vi "Enertool final com fecho do dia.vi"() -> ()   [LabVIEW 2017]
uses:
  System.Windows.Forms
  <vilib>/addons/database/Connection.llb/DB Tools Open Connec (Path).vi
  <vilib>/addons/database/NI_Database_API.lvlib
panel:
  out "?":string
  in  "OApa 3":bool
  in  "OK Hora 2":bool
  out "Array 2":string[][](array[string])
  in  "OK Hora Mes 2":bool
  in  "?":bool
  in  "OK Hora Mes":bool
  out "Array":string[][](array[string])
  in  "stop":bool
  out "TabGeral":T1(tab)
  in  "Login":string
  in  "?":bool
  in  "Zapcine":bool
  in  "Banco Bic":bool
  in  "wammo":bool
  in  "Candando":bool
  in  "MENU":bool
  out "Tab Control":enum32{"ONLINE", "REPORT"}(tab)
  out "PT Hiper - Contagem Energia Reactiva GG":string
  out "PT Hiper - Energia Reactiva Total (MWh)":string
  out "PT Hiper - Energia Activa Total":string
  out "PT Hiper - Contagem Energia GG":string
  out "PT Hiper - Contagem Energia Rede":string
  out "PT Hiper - Contagem Energia Reactiva Rede":string
  in  "REPORT":bool
  out "?":enum32{"DIARIO", "MENSAL", "ANUAL"}(tab)
  out "Total Mês":dbl[](graph)
  out "?":string
  out "?":string
  out "Total Mês":dbl[](graph)
  out "Ano":string
  in  "Month Calendar .NET Control":refnum<k24>(container)
  in  "Periodo":string(combo)
  in  "Pesquisar":bool
  out "Consumo Total (MWh)":dbl
  in  "ONLINE":bool
  in  "Combo Box":string(combo)="Contagem de Energia Reactiva GG"
  out "Tab Control 2":enum32{"ONLINE", "REPORT"}(tab)
  out "PT Cinemas - Contagem Energia Rede":string
  out "PT Cinemas - Contagem Energia GG":string
  out "PT Cinemas - Energia Activa Total":string
  out "PT Cinemas - Energia Reactiva Total (MWh)":string
  out "PT Cinemas - Contagem Energia Reactiva Rede":string
  out "PT Cinemas - Contagem Energia Reactiva GG":string
  in  "REPORT 2":bool
  out "?":enum32{"DIARIO", "MENSAL", "ANUAL"}(tab)
  out "Total Mês":dbl[](graph)
  out "?":string
  out "?":string
  out "Total Mês":dbl[](graph)
  out "Ano 2":string
  in  "Month Calendar .NET Control 2":refnum<k24>(container)
  in  "Periodo 2":string(combo)
  in  "Pesquisar 2":bool
  out "Consumo Total (MWh) 2":dbl
  in  "Combo Box 2":string(combo)="Contagem de Energia Reactiva GG"
  in  "MENU 2":bool
  in  "OK Hora":bool
  in  "OApa 2":bool
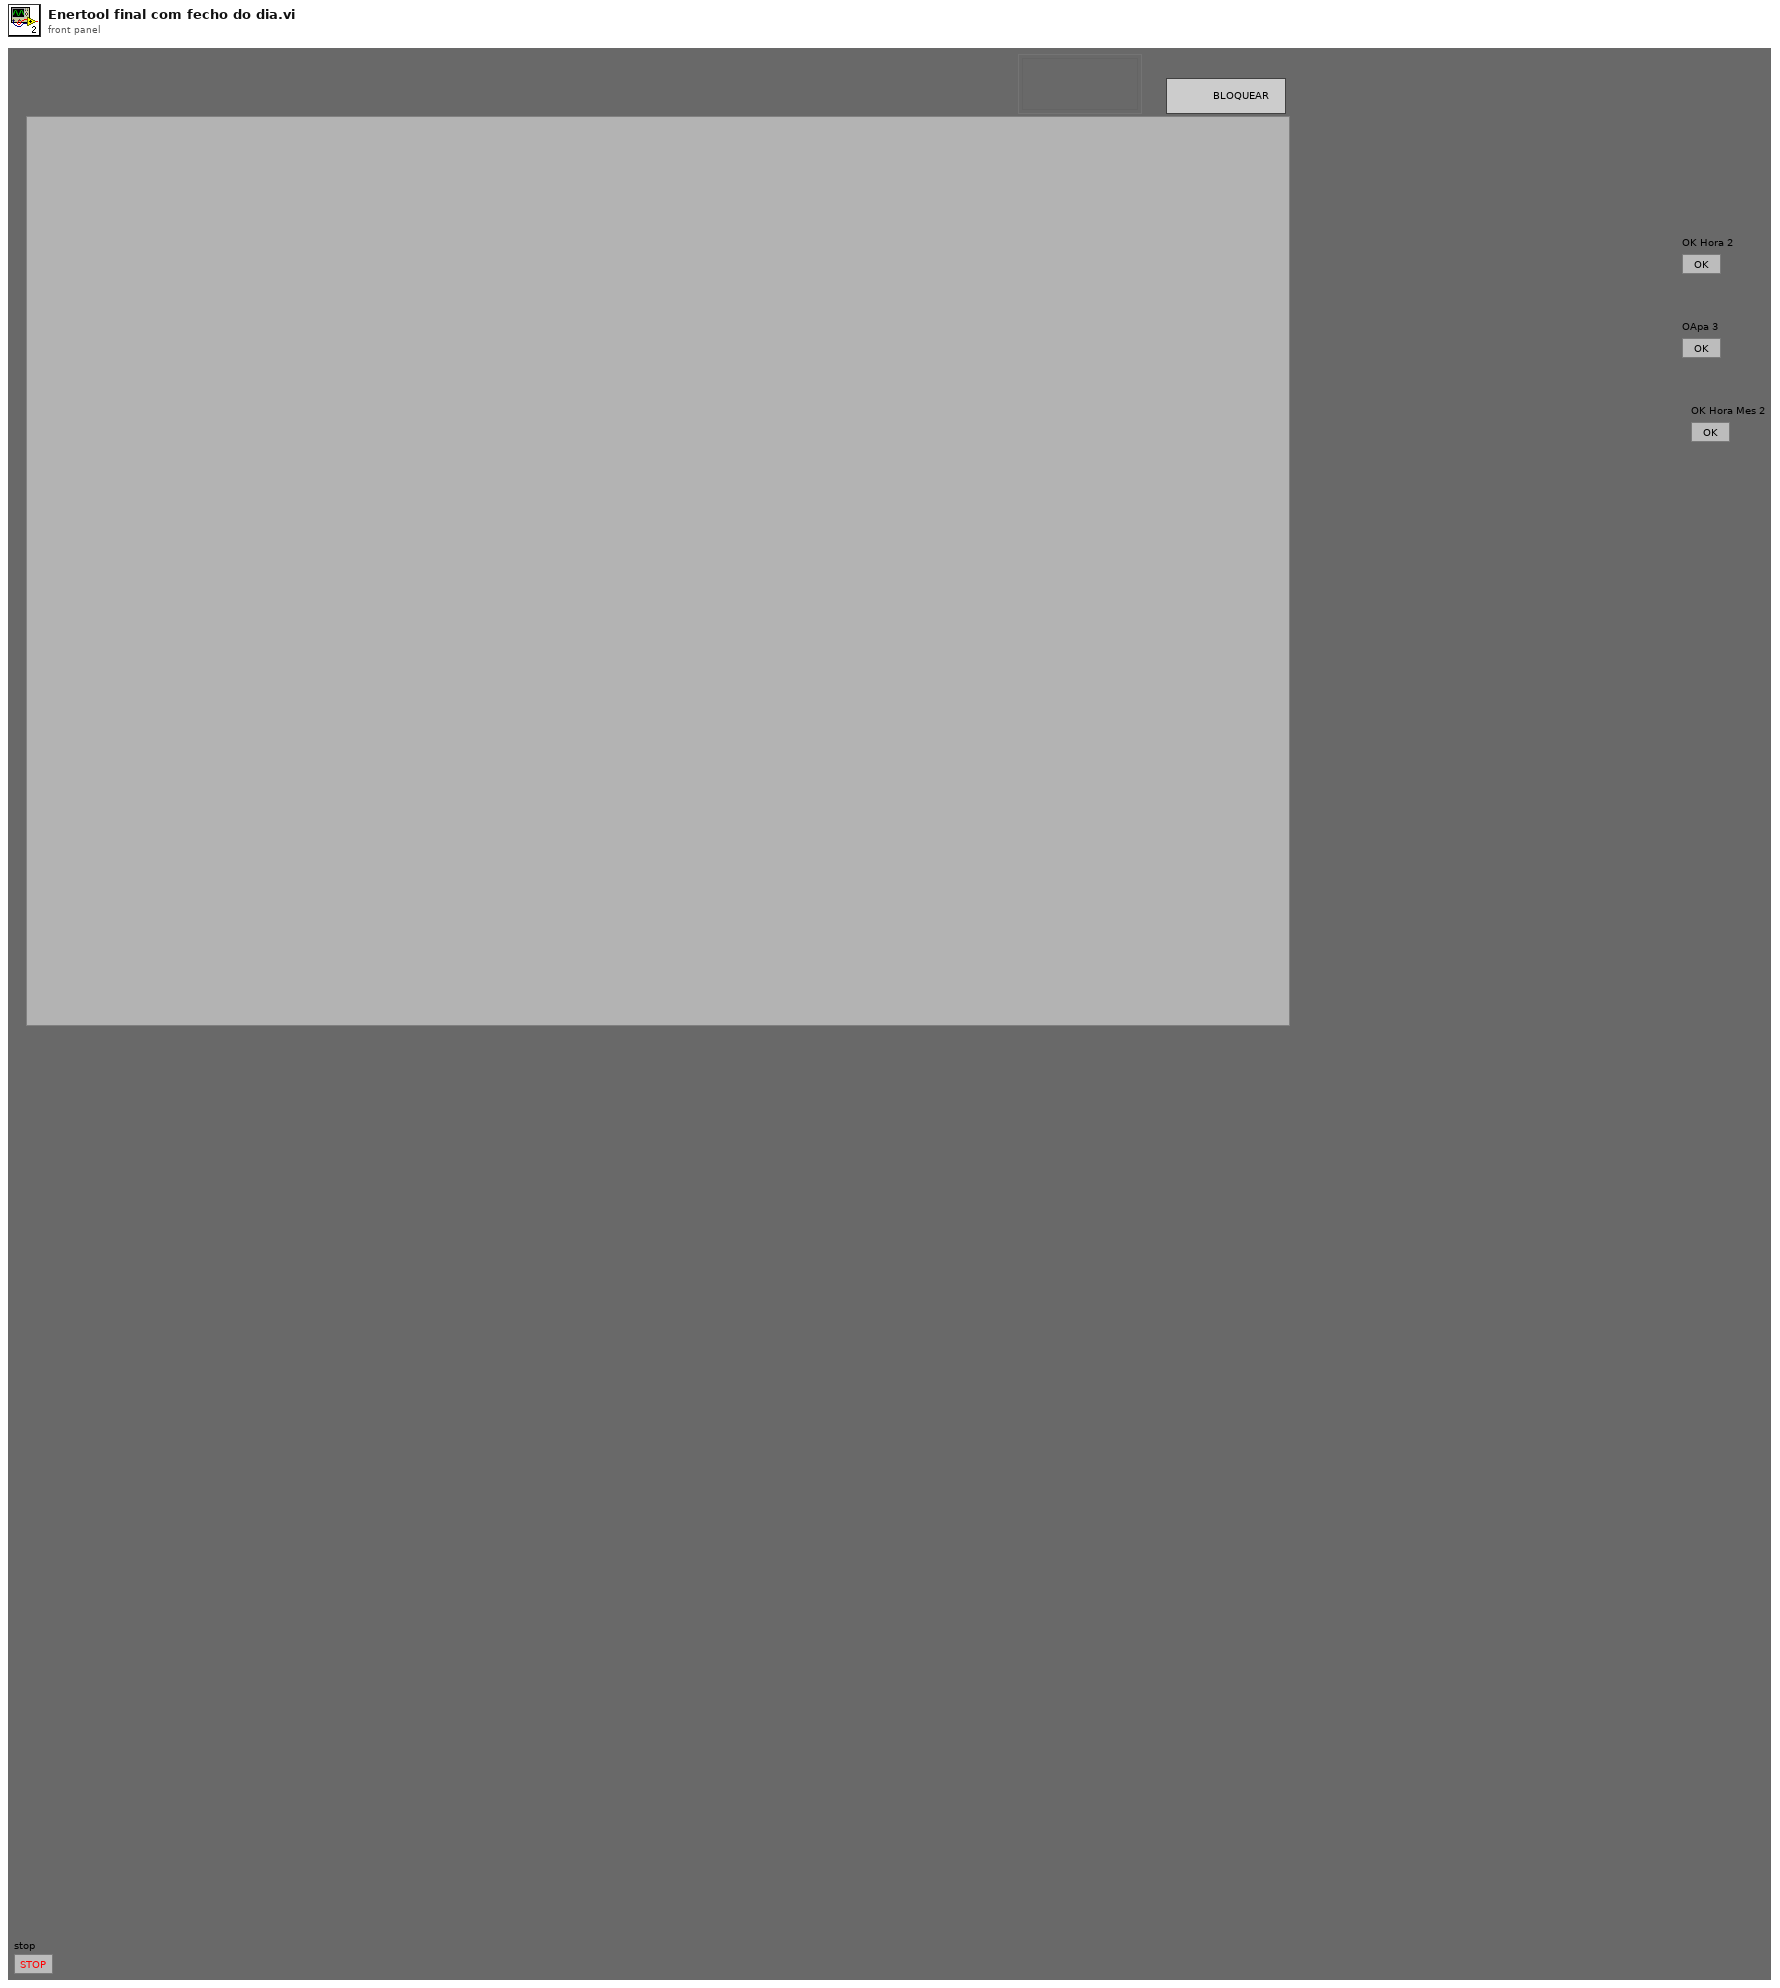
[diagram p1: front panel]
types:
  T1 = enum32{"Inicial", "Login", "Avennida", "HiperCandado", "ZapCinenma"}
  T2 = typedef "NI_Database_API.lvlib/Conn ObjectReference.ctl" = refnum<k1>
  T3 = enum16{"open", "replace", "create", "open or create", "replace or create", "replace or create with confirmation"}
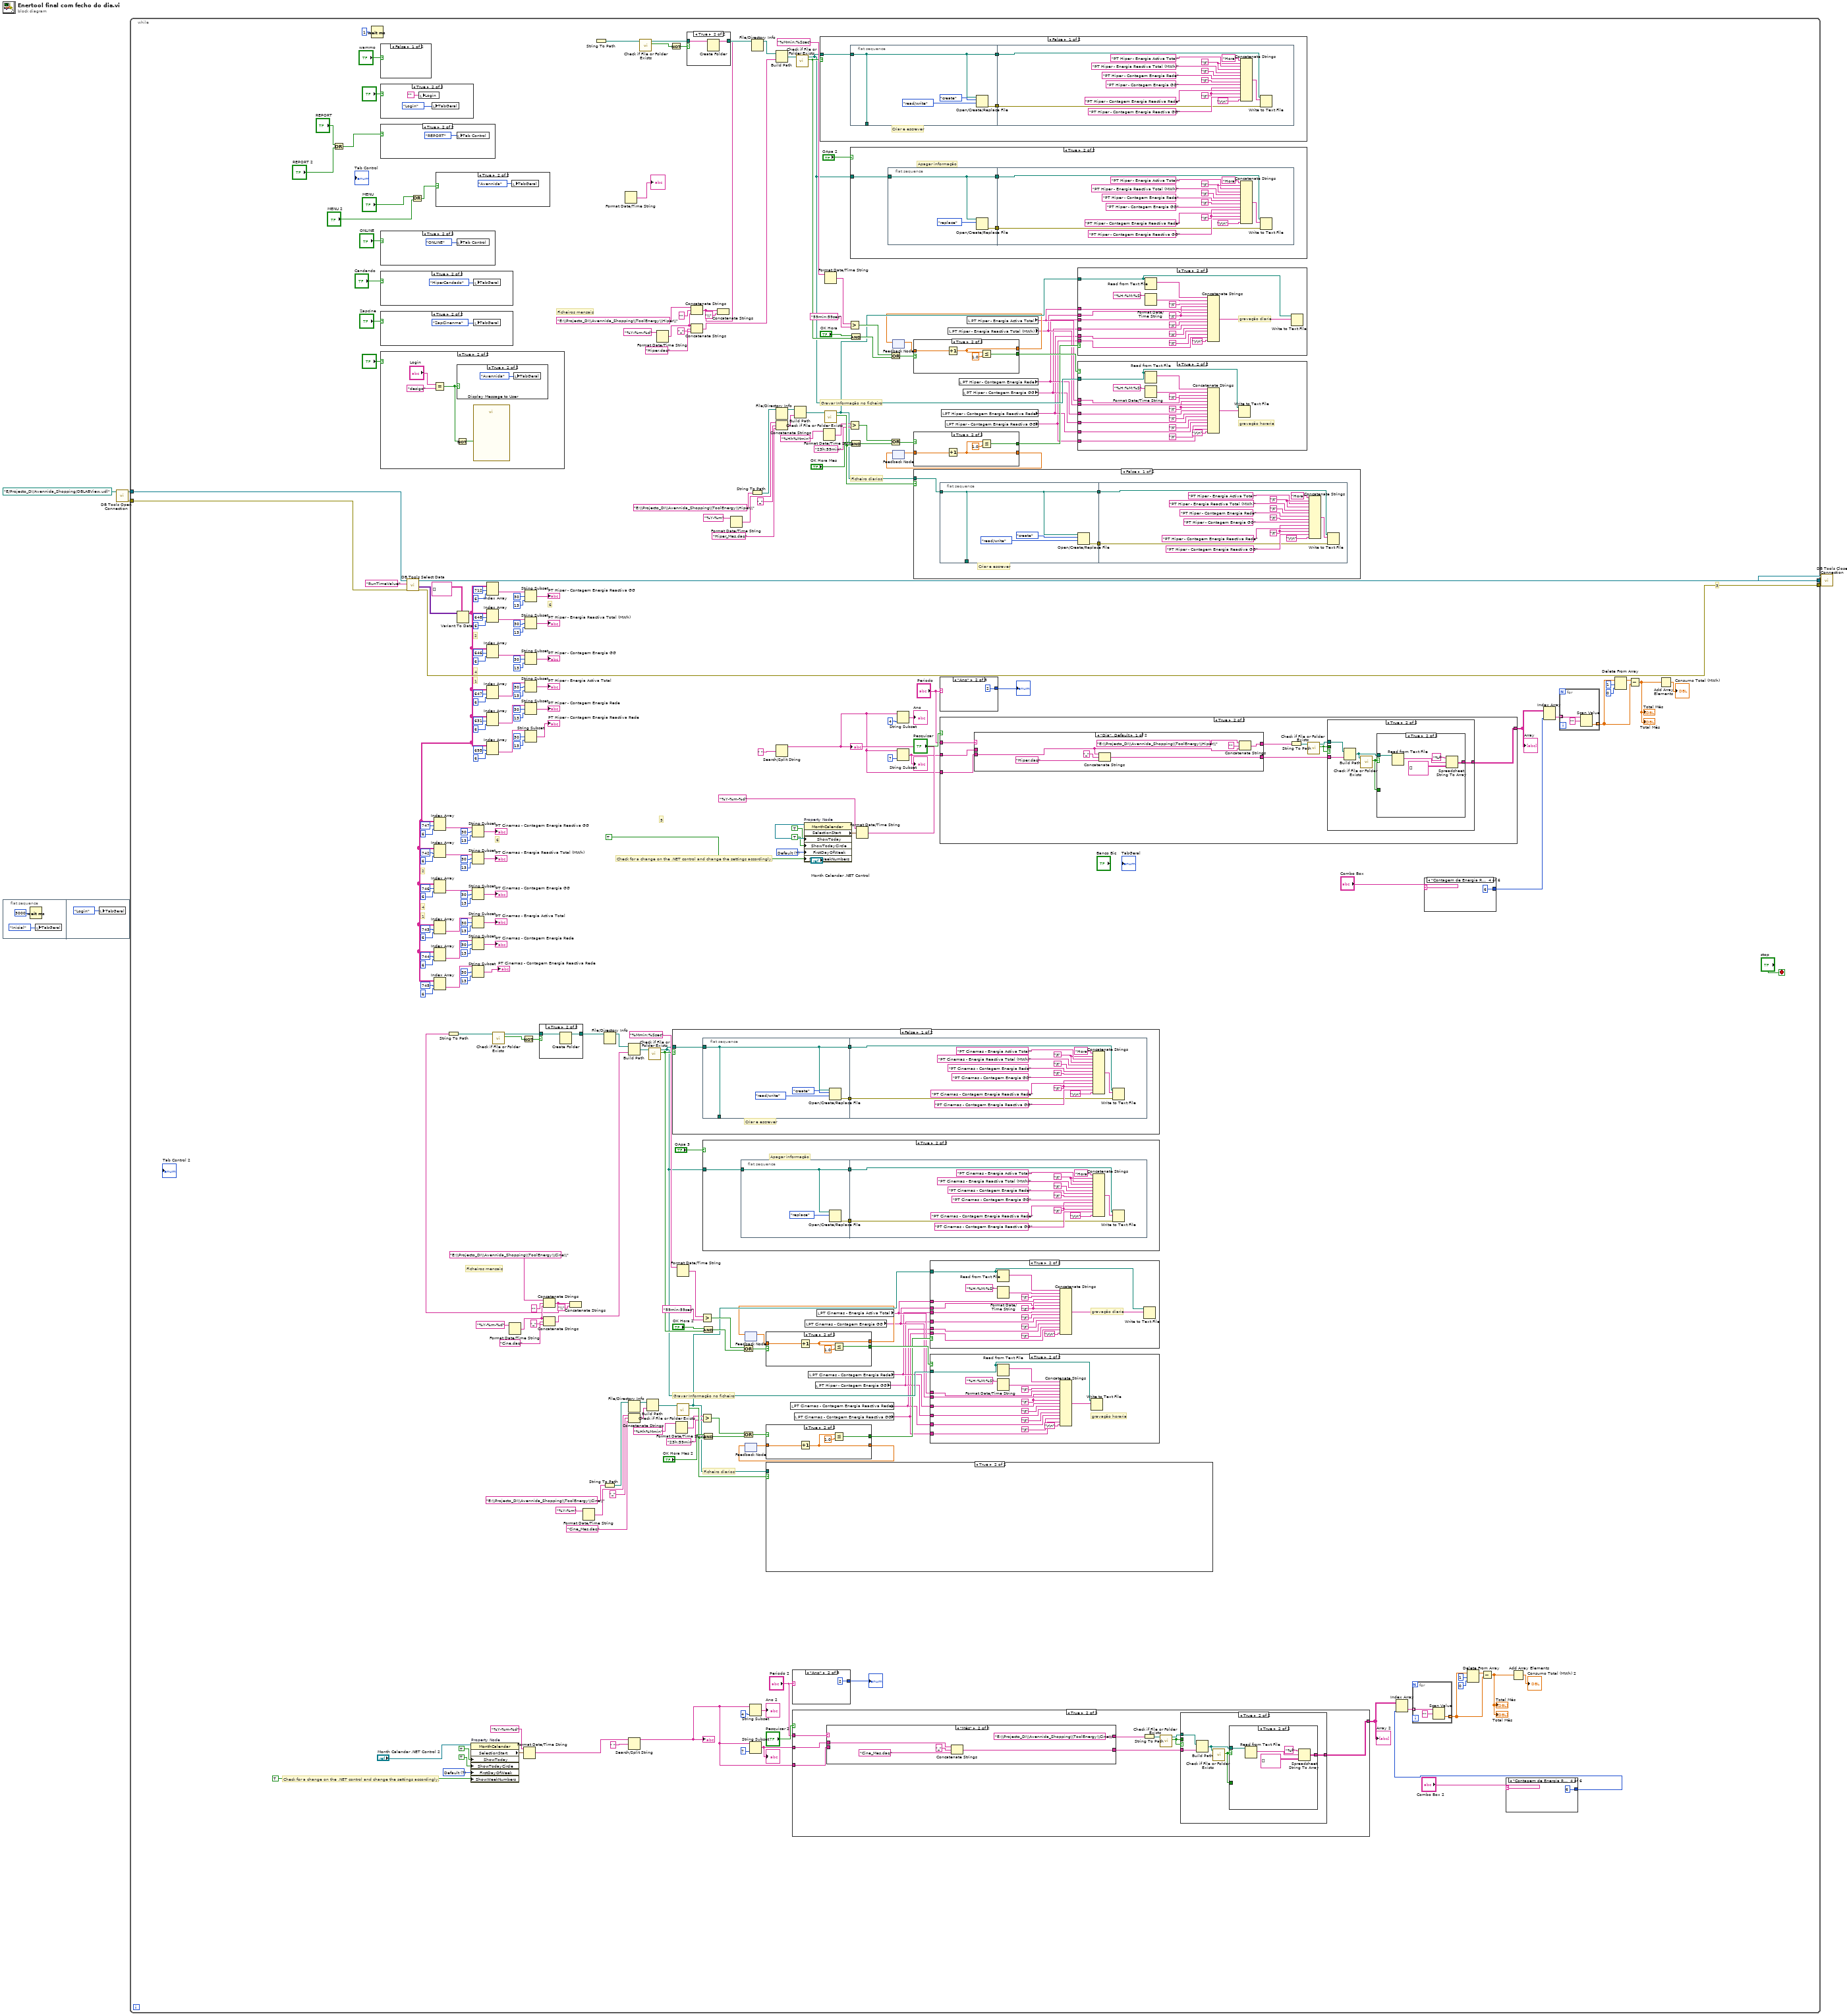
[diagram p0: block diagram]
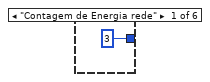
[diagram p2: hidden frame]
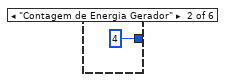
[diagram p3: hidden frame]
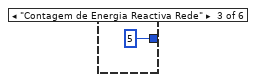
[diagram p4: hidden frame]
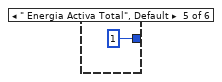
[diagram p5: hidden frame]
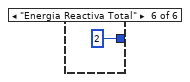
[diagram p6: hidden frame]
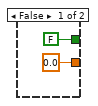
[diagram p7: hidden frame]
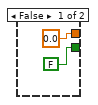
[diagram p8: hidden frame]
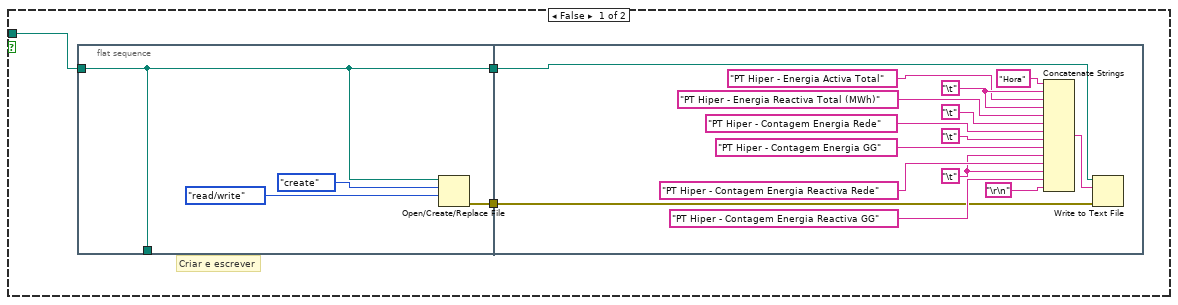
[diagram p11: hidden frame]
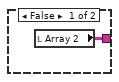
[diagram p14: hidden frame]
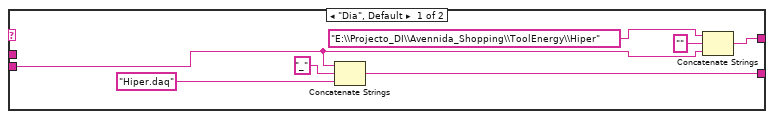
[diagram p15: hidden frame]
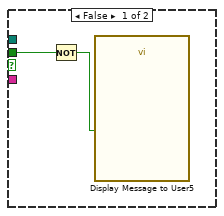
[diagram p16: hidden frame]
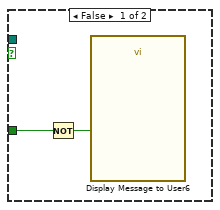
[diagram p17: hidden frame]
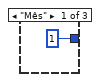
[diagram p18: hidden frame]
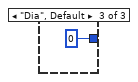
[diagram p19: hidden frame]
diagram:
  n1 = flat-sequence {
    frame #0 {
      n2 = Wait (ms)(milliseconds to wait=u32 3000) -> ()  [unwired: 1 out]
      n3 = local write "TabGeral"(T1."Inicial" ("TabGeral")) -> ()
    }
    frame #1 {
      n4 = local write "TabGeral"(T1."Login" ("TabGeral")) -> ()
    }
  }
  n5 = call-poly <vilib>:"DB Tools Open Connection.vi"("connection information"=path "E:/Projecto_DI/Avennida_Shopping/DBLABView.udl") -> ("error out"=w4:errorcluster, "connection reference"=w3:T2)  [unwired: 7 in]
  n6 = while {
    tunnel: w4 -> [w173]
    tunnel: w3 -> [w172]
    tunnel: [w171] -> w2
    tunnel: [w170] -> w1
    stop <- "stop" stop-if-true
    w93 = 7 items=["Monday", "Tuesday", "Wednesday", "Thursday", "Friday", "Saturday", "Sunday", "Default"] ("First Day of Week")
    w264 = 7 items=["Monday", "Tuesday", "Wednesday", "Thursday", "Friday", "Saturday", "Sunday", "Default"] ("First Day of Week")
    # "Ficheiros mensais"
    # "Ficheiro diarios"
    # "Gravar Informação no ficheiro"
    # "Check for a change on the .NET control and change the settings accordingly."
    # "1"
    # "2"
    # "4"
    # "6"
    # "1"
    # "2"
    # "3"
    # "4"
    # "5"
    # "6"
    # "Ficheiros mensais"
    # "Ficheiro diarios"
    # "Gravar Informação no ficheiro"
    # "Check for a change on the .NET control and change the settings accordingly."
    n7 = Or(x="REPORT", y="REPORT 2") -> (x .or. y?=w15:bool)
    n8 = Wait (ms)(milliseconds to wait=u32 1) -> ()  [unwired: 1 out]
    n9 = case shown="False" "wammo" {
      frame False {
      }
      frame True {
      }
    }
    n10 = case shown="True" "?" {
      frame False {
      }
      frame True {
        n11 = local write "Login"("") -> ()
        n12 = local write "TabGeral"(T1."Login" ("TabGeral")) -> ()
      }
    }
    n13 = case shown="True" w15 {
      frame False {
      }
      frame True {
        n14 = local write "Tab Control"(enum32{"ONLINE", "REPORT"}."REPORT" ("Tab Control")) -> ()
      }
    }
    n15 = case shown="True" "ONLINE" {
      frame False {
      }
      frame True {
        n16 = local write "Tab Control"(enum32{"ONLINE", "REPORT"}."ONLINE" ("Tab Control")) -> ()
      }
    }
    n17 = case shown="True" "Candando" {
      frame False {
      }
      frame True {
        n18 = local write "TabGeral"(T1."HiperCandado" ("TabGeral")) -> ()
      }
    }
    n19 = case shown="True" "Zapcine" {
      frame False {
      }
      frame True {
        n20 = local write "TabGeral"(T1."ZapCinenma" ("TabGeral")) -> ()
      }
    }
    n21 = case shown="True" "?" {
      frame False {
      }
      frame True {
        n22 = Equal?(x="Login", y="desigo") -> (x = y?=w577:bool)
        n23 = Not(x=w577) -> (.not. x?=w578:bool)
        n24 = case shown="True" w577 {
          frame False {
          }
          frame True {
            n25 = local write "TabGeral"(T1."Avennida" ("TabGeral")) -> ()
          }
        }
        n26 = call "Display Message to User"("Enable"=w578) -> ()  [unwired: 9 in, 2 out]
      }
    }
    n27 = call <vilib>:"DB Tools Select Data.vi"("error in (no error)"=w173, "table"="RunTimeValue", "connection reference"=w172) -> ("error out"=w171:errorcluster, "data"=w186:variant[][], "connection reference out"=w170:T2)  [unwired: 3 in]
    n28 = Or(x="MENU", y="MENU 2") -> (x .or. y?=w10:bool)
    n29 = case shown="True" w10 {
      frame False {
      }
      frame True {
        n30 = local write "TabGeral"(T1."Avennida" ("TabGeral")) -> ()
      }
    }
    n31 = Variant To Data(type=string[][] [], Variant=w186) -> (data=w99:string[][])  [unwired: 1 in, 1 out]
    n32 = Index Array(array=w99, index (row)=747, index (col)=6 ("disabled index (col) 2")) -> (element=w114:string)
    n33 = Index Array(array=w99, index (row)=742, index (col)=6 ("disabled index (col) 3")) -> (element=w127:string)
    n34 = Index Array(array=w99, index (row)=746, index (col)=6 ("disabled index (col) 3")) -> (element=w123:string)
    n35 = Index Array(array=w99, index (row)=743, index (col)=6 ("disabled index (col) 4")) -> (element=w119:string)
    n36 = Index Array(array=w99, index (row)=744, index (col)=6 ("disabled index (col) 3")) -> (element=w134:string)
    n37 = Index Array(array=w99, index (row)=745, index (col)=6 ("disabled index (col)")) -> (element=w116:string)
    n38 = property on="Property Node" class="MonthCalendar"(reference="Month Calendar .NET Control 2", "ShowToday"=TRUE ("Show Today"), "ShowTodayCircle"=TRUE ("Show Today Circle"), "FirstDayOfWeek"=w93, "ShowWeekNumbers"=TRUE ("Show Week Numbers")) -> ("SelectionStart"=w95:timestamp)  [unwired: 1 in, 2 out]
    n39 = String Subset(string=w114, offset (0)=30, length (rest)=13 ("length (rest)")) -> (substring=→"PT Cinemas - Contagem Energia Reactiva GG":string)
    n40 = String Subset(string=w127, offset (0)=30, length (rest)=13 ("length (rest)")) -> (substring=→"PT Cinemas - Energia Reactiva Total (MWh)":string)
    n41 = String Subset(string=w123, offset (0)=30, length (rest)=13 ("length (rest)")) -> (substring=→"PT Cinemas - Contagem Energia GG":string)
    n42 = String Subset(string=w119, offset (0)=30, length (rest)=13 ("length (rest)")) -> (substring=→"PT Cinemas - Energia Activa Total":string)
    n43 = String Subset(string=w134, offset (0)=30, length (rest)=13 ("length (rest)")) -> (substring=→"PT Cinemas - Contagem Energia Rede":string)
    n44 = String Subset(string=w116, offset (0)=30, length (rest)=13 ("length (rest)")) -> (substring=→"PT Cinemas - Contagem Energia Reactiva Rede":string)
    n45 = Index Array(array=w99, index (row)=712, index (col)=6 ("disabled index (col) 2")) -> (element=w165:string)
    n46 = Index Array(array=w99, index (row)=648, index (col)=6 ("disabled index (col) 3")) -> (element=w152:string)
    n47 = Index Array(array=w99, index (row)=646, index (col)=6 ("disabled index (col) 3")) -> (element=w156:string)
    n48 = Index Array(array=w99, index (row)=647, index (col)=6 ("disabled index (col) 4")) -> (element=w160:string)
    n49 = Index Array(array=w99, index (row)=631, index (col)=6 ("disabled index (col) 3")) -> (element=w145:string)
    n50 = Index Array(array=w99, index (row)=695, index (col)=6 ("disabled index (col)")) -> (element=w163:string)
    n51 = Format Date/Time String(time format string (%c)="%Y-%m-%d") -> (date/time string=w59:string)  [unwired: 2 in]
    n52 = Format Date/Time String(time format string (%c)="%Y-%m-%d", seconds (now)=w95) -> (date/time string=w94:string)  [unwired: 1 in]
    n53 = String Subset(string=w165, offset (0)=30, length (rest)=13 ("length (rest)")) -> (substring=→"PT Hiper - Contagem Energia Reactiva GG":string)
    n54 = String Subset(string=w152, offset (0)=30, length (rest)=13 ("length (rest)")) -> (substring=→"PT Hiper - Energia Reactiva Total (MWh)":string)
    n55 = String Subset(string=w156, offset (0)=30, length (rest)=13 ("length (rest)")) -> (substring=→"PT Hiper - Contagem Energia GG":string)
    n56 = String Subset(string=w160, offset (0)=30, length (rest)=13 ("length (rest)")) -> (substring=→"PT Hiper - Energia Activa Total":string)
    n57 = String Subset(string=w145, offset (0)=30, length (rest)=13 ("length (rest)")) -> (substring=→"PT Hiper - Contagem Energia Rede":string)
    n58 = String Subset(string=w163, offset (0)=30, length (rest)=13 ("length (rest)")) -> (substring=→"PT Hiper - Contagem Energia Reactiva Rede":string)
    n59 = Concatenate Strings("E:\\Projecto_DI\\Avennida_Shopping\\ToolEnergy\\Cine\\", "" ("string"), w59) -> (w48:string)
    n60 = String To Path(string=w48) -> (path=w50:path)
    n61 = call <vilib>:"Check if File or Folder Exists.vi"("path"=w50) -> ("file or folder exists?"=w52:bool, "dup path"=w51:path)  [unwired: 8 in, 1 out]
    n62 = Not(x=w52) -> (.not. x?=w53:bool)
    n63 = case shown="True" w53 {
      tunnel: w51 -> [w366 w368]
      tunnel: [w366 w367] -> w54
      frame False {
      }
      frame True {
        n64 = Create Folder(path (use dialog)=w368) -> (created path=w367:path)  [unwired: 2 in, 2 out]
      }
    }
    n65 = Concatenate Strings(w59, "_" ("string"), "Cine.daq" ("name or relative path")) -> (w58:string)
    n66 = Concatenate Strings(w48, "\\") -> ()  [unwired: 1 out]
    n67 = Format Date/Time String(time format string (%c)="%Y-%m") -> (date/time string=w43:string)  [unwired: 2 in]
    n68 = String To Path(string="E:\\Projecto_DI\\Avennida_Shopping\\ToolEnergy\\Cine\\") -> (path=w37:path)
    n69 = File/Directory Info(path=w54) -> (path out=w55:path)  [unwired: 1 in, 6 out]
    n70 = Format Date/Time String() -> (date/time string=→"?":string)  [unwired: 3 in]
    n71 = Build Path(base path=w55, name or relative path=w58) -> (appended path=w56:path)
    n72 = File/Directory Info(path=w37) -> (path out=w39:path)  [unwired: 1 in, 6 out]
    n73 = Concatenate Strings(w43, "_" ("string"), "Cine_Mes.daq" ("name or relative path")) -> (w42:string)
    n74 = Search/Split String(string=w94, search string/char (-)=" ") -> (substring before match=w83:string)  [unwired: 1 in, 2 out]
    "?" <- w83
    n75 = Build Path(base path=w39, name or relative path=w42) -> (appended path=w40:path)
    n76 = call <vilib>:"Check if File or Folder Exists.vi"("path"=w56) -> ("file or folder exists?"=w46:bool, "dup path"=w45:path)  [unwired: 8 in, 1 out]
    n77 = Format Date/Time String(time format string (%c)="%Y-%m-%d") -> (date/time string=w223:string)  [unwired: 2 in]
    n78 = case shown="False" w46 {
      tunnel: w45 -> [w346 _]
      frame False {
        # "Criar e escrever"
        n79 = flat-sequence {
          tunnel: w346 -> [w348]
          tunnel: [w348] -> _
          tunnel: [w348] -> w345
          tunnel: [w347] -> w344
          tunnel: w345 -> [w351]
          tunnel: w344 -> [w352]
          frame #0 {
            n80 = Open/Create/Replace File(file path (use dialog)=w348, operation (0:open)=T3."create", access (0:read/write)=enum16{"read/write", "read-only", "write-only"}."read/write") -> (error out=w347:errorcluster)  [unwired: 3 in, 2 out]
          }
          frame #1 {
            w362 = "\t"
            w355 = "\t"
            n81 = Concatenate Strings("Hora" ("string"), w355, "PT Cinemas - Energia Activa Total" ("string"), w355, "PT Cinemas - Energia Reactiva Total (MWh)" ("string"), "\t", "PT Cinemas - Contagem Energia Rede" ("string"), "\t", "PT Cinemas - Contagem Energia GG" ("string"), w362, "PT Cinemas - Contagem Energia Reactiva Rede" ("string"), w362, "PT Cinemas - Contagem Energia Reactiva GG" ("string"), "\r\n") -> (w353:string)
            n82 = Write to Text File(file (use dialog)=w351, text=w353, error in=w352) -> ()  [unwired: 1 in, 3 out]
          }
        }
      }
      frame True {
      }
    }
    n83 = Format Date/Time String(time format string (%c)="%Hh%Mmin") -> (date/time string=w67:string)  [unwired: 2 in]
    n84 = call <vilib>:"Check if File or Folder Exists.vi"("path"=w40) -> ("file or folder exists?"=w73:bool, "dup path"=w35:path)  [unwired: 8 in, 1 out]
    n85 = Format Date/Time String(time format string (%c)="%Mmin:%Ssec") -> (date/time string=w71:string)  [unwired: 2 in]
    n86 = Concatenate Strings("E:\\Projecto_DI\\Avennida_Shopping\\ToolEnergy\\Hiper\\", "" ("string"), w223) -> (w212:string)
    n87 = String To Path(string=w212) -> (path=w214:path)
    n88 = call <vilib>:"Check if File or Folder Exists.vi"("path"=w214) -> ("file or folder exists?"=w216:bool, "dup path"=w215:path)  [unwired: 8 in, 1 out]
    n89 = Not(x=w216) -> (.not. x?=w217:bool)
    n90 = case shown="True" w217 {
      tunnel: w215 -> [w527 w529]
      tunnel: [w527 w528] -> w218
      frame False {
      }
      frame True {
        n91 = Create Folder(path (use dialog)=w529) -> (created path=w528:path)  [unwired: 2 in, 2 out]
      }
    }
    n92 = Concatenate Strings(w223, "_" ("string"), "Hiper.daq" ("name or relative path")) -> (w222:string)
    n93 = Greater?(x=w71, y="59min:59sec") -> (0:w68:bool)
    n94 = Greater?(x=w67, y="23h:59min" ("y 2")) -> (0:w64:bool)
    n95 = And(x="OK Hora 2", y=w46) -> (x .and. y?=w69:bool)
    n96 = And(x="OK Hora Mes 2", y=w73) -> (x .and. y?=w65:bool)
    n97 = case shown="True" "OApa 3" {
      tunnel: w45 -> [_ w413]
      frame False {
      }
      frame True {
        # "Apagar informação"
        n98 = flat-sequence {
          tunnel: w413 -> [w414]
          tunnel: [w415] -> w412
          tunnel: [w414] -> w411
          tunnel: w412 -> [w418]
          tunnel: w411 -> [w417]
          frame #0 {
            n99 = Open/Create/Replace File(file path (use dialog)=w414, operation (0:open)=T3."replace") -> (error out=w415:errorcluster)  [unwired: 4 in, 2 out]
          }
          frame #1 {
            w422 = "\t"
            w429 = "\t"
            n100 = Concatenate Strings("Hora" ("string"), w429, "PT Cinemas - Energia Activa Total" ("string"), w429, "PT Cinemas - Energia Reactiva Total (MWh)" ("string"), "\t", "PT Cinemas - Contagem Energia Rede" ("string"), "\t", "PT Cinemas - Contagem Energia GG" ("string"), w422, "PT Cinemas - Contagem Energia Reactiva Rede" ("string"), w422, "PT Cinemas - Contagem Energia Reactiva GG" ("string"), "\r\n") -> (w431:string)
            n101 = Write to Text File(file (use dialog)=w417, text=w431, error in=w418) -> ()  [unwired: 1 in, 3 out]
          }
        }
      }
    }
    n102 = Concatenate Strings(w212, "\\") -> ()  [unwired: 1 out]
    n103 = Format Date/Time String(time format string (%c)="%Y-%m") -> (date/time string=w207:string)  [unwired: 2 in]
    n104 = Or(x=w68, y=w69) -> (x .or. y?=w32:bool)
    n105 = Or(x=w64, y=w65) -> (x .or. y?=w27:bool)
    n106 = feedback #1() -> (w33:dbl)  [unwired: 1 in]
    n107 = feedback #2() -> (w28:dbl)  [unwired: 1 in]
    n108 = String Subset(string=w83, length (rest)=4 ("length (rest)")) -> (substring=→"Ano 2":string)  [unwired: 1 in]
    n109 = String Subset(string=w83, length (rest)=7 ("length (rest)")) -> (substring=w25:string)  [unwired: 1 in]
    "?" <- w25
    n110 = String To Path(string="E:\\Projecto_DI\\Avennida_Shopping\\ToolEnergy\\Hiper\\") -> (path=w201:path)
    n111 = File/Directory Info(path=w218) -> (path out=w219:path)  [unwired: 1 in, 6 out]
    n112 = case shown="True" w32 {
      tunnel: [0.0 w284] -> w34
      tunnel: w33 -> [_ w287]
      tunnel: [FALSE w286] -> w31
      frame False {
      }
      frame True {
        n113 = Increment(x=w287) -> (x+1=w284:dbl)
        n114 = Less Or Equal?(x=w284, y=1.0) -> (x <= y?=w286:bool)
      }
    }
    n115 = feedback-in #1(w34) -> ()
    n116 = case shown="True" w27 {
      tunnel: [0.0 w279] -> w30
      tunnel: [FALSE w281] -> w29
      tunnel: w28 -> [_ w278]
      frame False {
      }
      frame True {
        n117 = Increment(x=w278) -> (x+1=w279:dbl)
        n118 = Less Or Equal?(x=w279, y=1.0) -> (x <= y?=w281:bool)
      }
    }
    n119 = feedback-in #2(w30) -> ()
    n120 = case shown="True" w73 {
      tunnel: w35 -> [w322 _]
      frame False {
        # "Criar e escrever"
        n121 = flat-sequence {
          tunnel: w322 -> [w326]
          tunnel: [w326] -> _
          tunnel: [w326] -> w324
          tunnel: [w325] -> w323
          tunnel: w324 -> [w333]
          tunnel: w323 -> [w332]
          frame #0 {
            n122 = Open/Create/Replace File(file path (use dialog)=w326, operation (0:open)=T3."create", access (0:read/write)=enum16{"read/write", "read-only", "write-only"}."read/write") -> (error out=w325:errorcluster)  [unwired: 3 in, 2 out]
          }
          frame #1 {
            w337 = "\t"
            w330 = "\t"
            n123 = Concatenate Strings("Hora" ("string"), w330, "PT Hiper - Energia Activa Total" ("string"), w330, "PT Hiper - Energia Reactiva Total (MWh)" ("string"), "\t", "PT Hiper - Contagem Energia Rede" ("string"), "\t", "PT Hiper - Contagem Energia GG" ("string"), w337, "PT Hiper - Contagem Energia Reactiva Rede" ("string"), w337, "PT Hiper - Contagem Energia Reactiva GG" ("string"), "\r\n") -> (w334:string)
            n124 = Write to Text File(file (use dialog)=w333, text=w334, error in=w332) -> ()  [unwired: 1 in, 3 out]
          }
        }
      }
      frame True {
      }
    }
    n125 = Build Path(base path=w219, name or relative path=w222) -> (appended path=w220:path)
    n126 = File/Directory Info(path=w201) -> (path out=w203:path)  [unwired: 1 in, 6 out]
    n127 = Concatenate Strings(w207, "_" ("string"), "Hiper_Mes.daq" ("name or relative path")) -> (w206:string)
    n128 = local read "PT Cinemas - Contagem Energia Reactiva Rede"() -> (w19:string)
    n129 = case shown="\"Ano\"" "Periodo 2" {
      tunnel: [1 2 0] -> w85
      frame "Mês" {
      }
      frame "Ano" {
      }
      frame "Dia", Default {
      }
    }
    "?" <- w85
    n130 = case shown="True" "Pesquisar 2" {
      tunnel: w83 -> [_ w375]
      tunnel: [w369 w372] -> w81
      tunnel: "Periodo 2" -> [_ w371]
      tunnel: w25 -> [_ w370]
      frame False {
        n131 = local read "Array 2"() -> (w369:string[][])
      }
      frame True {
        n132 = case shown="\"Mês\"" w371 {
          tunnel: [w382 "E:\\Projecto_DI\\Avennida_Shopping\\ToolEnergy\\Cine\\"] -> w376
          tunnel: w375 -> [w380 _]
          tunnel: [w379 w388] -> w374
          tunnel: w370 -> [_ w386]
          frame "Dia", Default {
            n133 = Concatenate Strings(w380, "_" ("string"), "Hiper.daq" ("name or relative path")) -> (w379:string)
            n134 = Concatenate Strings("E:\\Projecto_DI\\Avennida_Shopping\\ToolEnergy\\Hiper", "" ("string"), w380) -> (w382:string)
          }
          frame "Mês" {
            n135 = Concatenate Strings(w386, "_" ("string"), "Cine_Mes.daq" ("name or relative path")) -> (w388:string)
          }
        }
        n136 = String To Path(string=w376) -> (path=w377:path)
        n137 = call <vilib>:"Check if File or Folder Exists.vi"("path"=w377) -> ("file or folder exists?"=w373:bool, "dup path"=w378:path)  [unwired: 8 in, 1 out]
        n138 = case shown="True" w373 {
          tunnel: w378 -> [_ w395]
          tunnel: w374 -> [_ w397]
          tunnel: w373 -> [w391 _]
          tunnel: [_ w394] -> w372
          frame False {
            n139 = Not(x=w391) -> (.not. x?=w392:bool)
            n140 = call "Display Message to User5"("Enable"=w392) -> ()  [unwired: 9 in, 2 out]
          }
          frame True {
            n141 = Build Path(base path=w395, name or relative path=w397) -> (appended path=w393:path)
            n142 = call <vilib>:"Check if File or Folder Exists.vi"("path"=w393) -> ("file or folder exists?"=w396:bool)  [unwired: 8 in, 2 out]
            n143 = case shown="True" w396 {
              tunnel: w396 -> [w398 _]
              tunnel: w393 -> [_ w401]
              tunnel: [_ w400] -> w394
              frame False {
                n144 = Not(x=w398) -> (.not. x?=w399:bool)
                n145 = call "Display Message to User6"("Enable"=w399) -> ()  [unwired: 9 in, 2 out]
              }
              frame True {
                n146 = Read from Text File(file (use dialog)=w401) -> (text=w404:string)  [unwired: 3 in, 3 out]
                n147 = Spreadsheet String To Array(format string="%f", spreadsheet string=w404, array type (2D Dbl)=string[][] [] ("Array")) -> (array=w400:string[][])  [unwired: 1 in]
              }
            }
          }
        }
      }
    }
    "Array 2" <- w81
    n148 = Build Path(base path=w203, name or relative path=w206) -> (appended path=w204:path)
    n149 = local read "PT Cinemas - Contagem Energia Reactiva GG"() -> (w18:string)
    n150 = call <vilib>:"Check if File or Folder Exists.vi"("path"=w220) -> ("file or folder exists?"=w210:bool, "dup path"=w209:path)  [unwired: 8 in, 1 out]
    n151 = property on="Property Node" class="MonthCalendar"(reference="Month Calendar .NET Control", "ShowToday"=TRUE ("Show Today"), "ShowTodayCircle"=TRUE ("Show Today Circle"), "FirstDayOfWeek"=w264, "ShowWeekNumbers"=TRUE ("Show Week Numbers")) -> ("SelectionStart"=w266:timestamp)  [unwired: 1 in, 2 out]
    n152 = local read "PT Cinemas - Contagem Energia GG"() -> (w22:string)
    n153 = local read "PT Cinemas - Contagem Energia Rede"() -> (w21:string)
    n154 = local read "PT Hiper - Contagem Energia GG"() -> (w20:string)
    n155 = local read "PT Cinemas - Energia Activa Total"() -> (w23:string)
    n156 = case shown="False" w210 {
      tunnel: w209 -> [w507 _]
      frame False {
        # "Criar e escrever"
        n157 = flat-sequence {
          tunnel: w507 -> [w509]
          tunnel: [w509] -> _
          tunnel: [w509] -> w506
          tunnel: [w508] -> w505
          tunnel: w506 -> [w512]
          tunnel: w505 -> [w513]
          frame #0 {
            n158 = Open/Create/Replace File(file path (use dialog)=w509, operation (0:open)=T3."create", access (0:read/write)=enum16{"read/write", "read-only", "write-only"}."read/write") -> (error out=w508:errorcluster)  [unwired: 3 in, 2 out]
          }
          frame #1 {
            w523 = "\t"
            w516 = "\t"
            n159 = Concatenate Strings("Hora" ("string"), w516, "PT Hiper - Energia Activa Total" ("string"), w516, "PT Hiper - Energia Reactiva Total (MWh)" ("string"), "\t", "PT Hiper - Contagem Energia Rede" ("string"), "\t", "PT Hiper - Contagem Energia GG" ("string"), w523, "PT Hiper - Contagem Energia Reactiva Rede" ("string"), w523, "PT Hiper - Contagem Energia Reactiva GG" ("string"), "\r\n") -> (w514:string)
            n160 = Write to Text File(file (use dialog)=w512, text=w514, error in=w513) -> ()  [unwired: 1 in, 3 out]
          }
        }
      }
      frame True {
      }
    }
    n161 = Format Date/Time String(time format string (%c)="%Hh%Mmin") -> (date/time string=w231:string)  [unwired: 2 in]
    n162 = call <vilib>:"Check if File or Folder Exists.vi"("path"=w204) -> ("file or folder exists?"=w237:bool, "dup path"=w199:path)  [unwired: 8 in, 1 out]
    n163 = Format Date/Time String(time format string (%c)="%Mmin:%Ssec") -> (date/time string=w235:string)  [unwired: 2 in]
    n164 = Greater?(x=w235, y="59min:59sec") -> (0:w232:bool)
    n165 = Greater?(x=w231, y="23h:59min" ("y 2")) -> (0:w228:bool)
    n166 = And(x="OK Hora", y=w210) -> (x .and. y?=w233:bool)
    n167 = And(x="OK Hora Mes", y=w237) -> (x .and. y?=w229:bool)
    n168 = case shown="True" "OApa 2" {
      tunnel: w209 -> [_ w587]
      frame False {
      }
      frame True {
        # "Apagar informação"
        n169 = flat-sequence {
          tunnel: w587 -> [w588]
          tunnel: [w589] -> w586
          tunnel: [w588] -> w585
          tunnel: w586 -> [w592]
          tunnel: w585 -> [w591]
          frame #0 {
            n170 = Open/Create/Replace File(file path (use dialog)=w588, operation (0:open)=T3."replace") -> (error out=w589:errorcluster)  [unwired: 4 in, 2 out]
          }
          frame #1 {
            w596 = "\t"
            w603 = "\t"
            n171 = Concatenate Strings("Hora" ("string"), w603, "PT Hiper - Energia Activa Total" ("string"), w603, "PT Hiper - Energia Reactiva Total (MWh)" ("string"), "\t", "PT Hiper - Contagem Energia Rede" ("string"), "\t", "PT Hiper - Contagem Energia GG" ("string"), w596, "PT Hiper - Contagem Energia Reactiva Rede" ("string"), w596, "PT Hiper - Contagem Energia Reactiva GG" ("string"), "\r\n") -> (w605:string)
            n172 = Write to Text File(file (use dialog)=w591, text=w605, error in=w592) -> ()  [unwired: 1 in, 3 out]
          }
        }
      }
    }
    n173 = Format Date/Time String(time format string (%c)="%Y-%m-%d", seconds (now)=w266) -> (date/time string=w265:string)  [unwired: 1 in]
    n174 = Search/Split String(string=w265, search string/char (-)=" ") -> (substring before match=w251:string)  [unwired: 1 in, 2 out]
    "?" <- w251
    n175 = Or(x=w232, y=w233) -> (x .or. y?=w196:bool)
    n176 = Or(x=w228, y=w229) -> (x .or. y?=w191:bool)
    n177 = feedback #3() -> (w197:dbl)  [unwired: 1 in]
    n178 = feedback #4() -> (w192:dbl)  [unwired: 1 in]
    n179 = String Subset(string=w251, length (rest)=4 ("length (rest)")) -> (substring=→"Ano":string)  [unwired: 1 in]
    n180 = String Subset(string=w251, length (rest)=7 ("length (rest)")) -> (substring=w189:string)  [unwired: 1 in]
    "?" <- w189
    n181 = case shown="True" w196 {
      tunnel: [0.0 w445] -> w198
      tunnel: w197 -> [_ w448]
      tunnel: [FALSE w447] -> w195
      frame False {
      }
      frame True {
        n182 = Increment(x=w448) -> (x+1=w445:dbl)
        n183 = Less Or Equal?(x=w445, y=1.0) -> (x <= y?=w447:bool)
      }
    }
    n184 = feedback-in #3(w198) -> ()
    n185 = case shown="True" w191 {
      tunnel: [0.0 w440] -> w194
      tunnel: [FALSE w442] -> w193
      tunnel: w192 -> [_ w439]
      frame False {
      }
      frame True {
        n186 = Increment(x=w439) -> (x+1=w440:dbl)
        n187 = Less Or Equal?(x=w440, y=1.0) -> (x <= y?=w442:bool)
      }
    }
    n188 = feedback-in #4(w194) -> ()
    n189 = case shown="False" w237 {
      tunnel: w199 -> [w483 _]
      frame False {
        # "Criar e escrever"
        n190 = flat-sequence {
          tunnel: w483 -> [w487]
          tunnel: [w487] -> _
          tunnel: [w487] -> w485
          tunnel: [w486] -> w484
          tunnel: w485 -> [w494]
          tunnel: w484 -> [w493]
          frame #0 {
            n191 = Open/Create/Replace File(file path (use dialog)=w487, operation (0:open)=T3."create", access (0:read/write)=enum16{"read/write", "read-only", "write-only"}."read/write") -> (error out=w486:errorcluster)  [unwired: 3 in, 2 out]
          }
          frame #1 {
            w498 = "\t"
            w491 = "\t"
            n192 = Concatenate Strings("Hora" ("string"), w491, "PT Hiper - Energia Activa Total" ("string"), w491, "PT Hiper - Energia Reactiva Total (MWh)" ("string"), "\t", "PT Hiper - Contagem Energia Rede" ("string"), "\t", "PT Hiper - Contagem Energia GG" ("string"), w498, "PT Hiper - Contagem Energia Reactiva Rede" ("string"), w498, "PT Hiper - Contagem Energia Reactiva GG" ("string"), "\r\n") -> (w495:string)
            n193 = Write to Text File(file (use dialog)=w494, text=w495, error in=w493) -> ()  [unwired: 1 in, 3 out]
          }
        }
      }
      frame True {
      }
    }
    n194 = case shown="True" w29 {
      tunnel: w23 -> [_ w295]
      tunnel: w22 -> [_ w294]
      tunnel: w21 -> [_ w293]
      tunnel: w20 -> [_ w292]
      tunnel: w19 -> [_ w291]
      tunnel: w18 -> [_ w290]
      tunnel: w35 -> [_ w288]
      frame False {
      }
      frame True {
        w303 = "\t"
        # "gravação diaria"
        n195 = Read from Text File(file (use dialog)=w288) -> (text=w289:string)  [unwired: 3 in, 3 out]
        n196 = Format Date/Time String(time format string (%c)="%H:%M:%S") -> (date/time string=w302:string)  [unwired: 2 in]
        n197 = Concatenate Strings(w289, w302, "\t", w295, w303, w294, w303, w293, "\t", w292, "\t", w291, "\t", w290, "\r\n") -> (w296:string)
        n198 = Write to Text File(file (use dialog)=w288, text=w296) -> ()  [unwired: 2 in, 3 out]
      }
    }
    n199 = case shown="True" w31 {
      tunnel: w22 -> [_ w321]
      tunnel: w21 -> [_ w320]
      tunnel: w20 -> [_ w318]
      tunnel: w19 -> [_ w316]
      tunnel: w18 -> [_ w314]
      tunnel: w23 -> [_ w312]
      tunnel: w45 -> [_ w306]
      frame False {
      }
      frame True {
        w308 = "\t"
        # "gravação horaria"
        n200 = Read from Text File(file (use dialog)=w306) -> (text=w309:string)  [unwired: 3 in, 3 out]
        n201 = Format Date/Time String(time format string (%c)="%H:%M:%S") -> (date/time string=w310:string)  [unwired: 2 in]
        n202 = Concatenate Strings(w309, w310, "\t", w312, w308, w321, w308, w320, "\t", w318, "\t", w316, "\t", w314, "\r\n") -> (w305:string)
        n203 = Write to Text File(file (use dialog)=w306, text=w305) -> ()  [unwired: 2 in, 3 out]
      }
    }
    n204 = case shown="\"Ano\"" "Periodo" {
      tunnel: [1 2 0] -> w256
      frame "Mês" {
      }
      frame "Ano" {
      }
      frame "Dia", Default {
      }
    }
    "?" <- w256
    n205 = case shown="True" "Pesquisar" {
      tunnel: w251 -> [_ w538]
      tunnel: [w532 w535] -> w249
      tunnel: "Periodo" -> [_ w534]
      tunnel: w189 -> [_ w533]
      frame False {
        n206 = local read "Array"() -> (w532:string[][])
      }
      frame True {
        n207 = case shown="\"Dia\", Default" w534 {
          tunnel: [w545 "E:\\Projecto_DI\\Avennida_Shopping\\ToolEnergy\\Hiper\\"] -> w539
          tunnel: w538 -> [w543 _]
          tunnel: [w542 w551] -> w537
          tunnel: w533 -> [_ w549]
          frame "Dia", Default {
            n208 = Concatenate Strings(w543, "_" ("string"), "Hiper.daq" ("name or relative path")) -> (w542:string)
            n209 = Concatenate Strings("E:\\Projecto_DI\\Avennida_Shopping\\ToolEnergy\\Hiper\\", "" ("string"), w543) -> (w545:string)
          }
          frame "Mês" {
            n210 = Concatenate Strings(w549, "_" ("string"), "Hiper_Mes.daq" ("name or relative path")) -> (w551:string)
          }
        }
        n211 = String To Path(string=w539) -> (path=w540:path)
        n212 = call <vilib>:"Check if File or Folder Exists.vi"("path"=w540) -> ("file or folder exists?"=w536:bool, "dup path"=w541:path)  [unwired: 8 in, 1 out]
        n213 = case shown="True" w536 {
          tunnel: w541 -> [_ w558]
          tunnel: w537 -> [_ w560]
          tunnel: w536 -> [w554 _]
          tunnel: [_ w557] -> w535
          frame False {
            n214 = Not(x=w554) -> (.not. x?=w555:bool)
            n215 = call "Display Message to User2"("Enable"=w555) -> ()  [unwired: 9 in, 2 out]
          }
          frame True {
            n216 = Build Path(base path=w558, name or relative path=w560) -> (appended path=w556:path)
            n217 = call <vilib>:"Check if File or Folder Exists.vi"("path"=w556) -> ("file or folder exists?"=w559:bool)  [unwired: 8 in, 2 out]
            n218 = case shown="True" w559 {
              tunnel: w559 -> [w561 _]
              tunnel: w556 -> [_ w564]
              tunnel: [_ w563] -> w557
              frame False {
                n219 = Not(x=w561) -> (.not. x?=w562:bool)
                n220 = call "Display Message to User3"("Enable"=w562) -> ()  [unwired: 9 in, 2 out]
              }
              frame True {
                n221 = Read from Text File(file (use dialog)=w564) -> (text=w567:string)  [unwired: 3 in, 3 out]
                n222 = Spreadsheet String To Array(format string="%f", spreadsheet string=w567, array type (2D Dbl)=string[][] [] ("Array")) -> (array=w563:string[][])  [unwired: 1 in]
              }
            }
          }
        }
      }
    }
    "Array" <- w249
    n223 = local read "PT Hiper - Contagem Energia Reactiva Rede"() -> (w139:string)
    n224 = local read "PT Hiper - Contagem Energia Reactiva GG"() -> (w138:string)
    n225 = local read "PT Hiper - Energia Reactiva Total (MWh)"() -> (w142:string)
    n226 = local read "PT Hiper - Contagem Energia Rede"() -> (w141:string)
    n227 = local read "PT Hiper - Contagem Energia GG"() -> (w140:string)
    n228 = local read "PT Hiper - Energia Activa Total"() -> (w143:string)
    n229 = case shown="True" w193 {
      tunnel: w143 -> [_ w456]
      tunnel: w142 -> [_ w455]
      tunnel: w141 -> [_ w454]
      tunnel: w140 -> [_ w453]
      tunnel: w139 -> [_ w452]
      tunnel: w138 -> [_ w451]
      tunnel: w199 -> [_ w449]
      frame False {
      }
      frame True {
        w464 = "\t"
        # "gravação diaria"
        n230 = Read from Text File(file (use dialog)=w449) -> (text=w450:string)  [unwired: 3 in, 3 out]
        n231 = Format Date/Time String(time format string (%c)="%H:%M:%S") -> (date/time string=w463:string)  [unwired: 2 in]
        n232 = Concatenate Strings(w450, w463, "\t", w456, w464, w455, w464, w454, "\t", w453, "\t", w452, "\t", w451, "\r\n") -> (w457:string)
        n233 = Write to Text File(file (use dialog)=w449, text=w457) -> ()  [unwired: 2 in, 3 out]
      }
    }
    n234 = case shown="True" w195 {
      tunnel: w142 -> [_ w482]
      tunnel: w141 -> [_ w481]
      tunnel: w140 -> [_ w479]
      tunnel: w139 -> [_ w477]
      tunnel: w138 -> [_ w475]
      tunnel: w143 -> [_ w473]
      tunnel: w209 -> [_ w467]
      frame False {
      }
      frame True {
        w469 = "\t"
        # "gravação horaria"
        n235 = Read from Text File(file (use dialog)=w467) -> (text=w470:string)  [unwired: 3 in, 3 out]
        n236 = Format Date/Time String(time format string (%c)="%H:%M:%S") -> (date/time string=w471:string)  [unwired: 2 in]
        n237 = Concatenate Strings(w470, w471, "\t", w473, w469, w482, w469, w481, "\t", w479, "\t", w477, "\t", w475, "\r\n") -> (w466:string)
        n238 = Write to Text File(file (use dialog)=w467, text=w466) -> ()  [unwired: 2 in, 3 out]
      }
    }
    n239 = case shown="\"Contagem de Energia Reactiva GG\"" "Combo Box" {
      tunnel: [3 4 5 6 1 2] -> w254
      frame "Contagem de Energia rede" {
      }
      frame "Contagem de Energia Gerador" {
      }
      frame "Contagem de Energia Reactiva Rede" {
      }
      frame "Contagem de Energia Reactiva GG" {
      }
      frame " Energia Activa Total", Default {
      }
      frame "Energia Reactiva Total" {
      }
    }
    n240 = case shown="\"Contagem de Energia Reactiva GG\"" "Combo Box 2" {
      tunnel: [3 4 5 6 1 2] -> w16
      frame "Contagem de Energia rede" {
      }
      frame "Contagem de Energia Gerador" {
      }
      frame "Contagem de Energia Reactiva Rede" {
      }
      frame "Contagem de Energia Reactiva GG" {
      }
      frame " Energia Activa Total", Default {
      }
      frame "Energia Reactiva Total" {
      }
    }
    n241 = Index Array(array=w81, index (col)=w16) -> (element=w84:string[])  [unwired: 1 in]
    n242 = for {
      tunnel: w84 -> [w407] mode=indexing
      tunnel: [w406] -> w77 mode=indexing
      n243 = Scan Value(string=w407, format string="") -> (value=w406:dbl)  [unwired: 1 in, 1 out]
    }
    n244 = Delete From Array(array=w77, length=1, index=0) -> (array with subset deleted=w78:dbl[])  [unwired: 1 out]
    n245 = Subtract(x=w78, y=w77) -> (x-y=w24:dbl[])
    "Total Mês" <- w24
    "Total Mês" <- w24
    n246 = Add Array Elements(numeric array=w24) -> (sum=→"Consumo Total (MWh) 2":dbl)
    n247 = Index Array(array=w249, index (col)=w254) -> (element=w253:string[])  [unwired: 1 in]
    n248 = for {
      tunnel: w253 -> [w576] mode=indexing
      tunnel: [w575] -> w241 mode=indexing
      n249 = Scan Value(string=w576, format string="") -> (value=w575:dbl)  [unwired: 1 in, 1 out]
    }
    n250 = Delete From Array(array=w241, length=1, index=0) -> (array with subset deleted=w242:dbl[])  [unwired: 1 out]
    n251 = Subtract(x=w242, y=w241) -> (x-y=w188:dbl[])
    "Total Mês" <- w188
    "Total Mês" <- w188
    n252 = Add Array Elements(numeric array=w188) -> (sum=→"Consumo Total (MWh)":dbl)
  }
  n253 = call <vilib>:"DB Tools Close Connection.vi"("error in (no error)"=w2, "connection reference"=w1) -> ()  [unwired: 5 in, 1 out]
